vi "Actual Sample Mode.vi"(8 "error in (no error)":errorcluster {"code" format="%.0x"}, 11 "VISA Resource Name":refnum<visa-resource-name>) -> (0 "error out":errorcluster {"code" format="%.0x"}, 2 "Sample Mode":i32(ring)=1 items=["Real Time", "Equivalent Time"], 3 "VISA Resource Name Out":refnum<visa-resource-name>)   [LabVIEW 2010, in "Tektronix TDS 3000 Series.lvlib"]
doc: "This VI returns the sample mode the oscilloscope is currently using."
uses:
  <instrlib>/Tektronix TDS 3000 Series/Tektronix TDS 3000 Series.lvlib
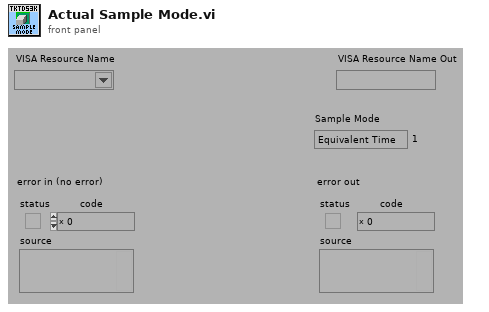
[diagram p1: front panel]
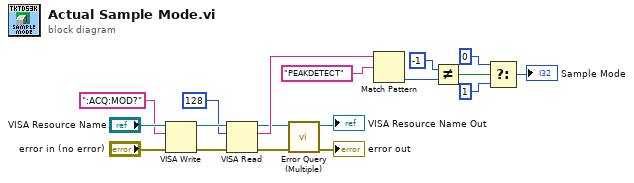
[diagram p0: block diagram]
diagram:
  n1 = VISA Write(VISA resource name="VISA Resource Name", write buffer=":ACQ:MOD?", error in (no error)="error in (no error)") -> (VISA resource name out=w18:refnum<visa-resource-name>, error out=w17:errorcluster)  [unwired: 1 out]
  n2 = VISA Read(VISA resource name=w18, byte count=u32 128, error in (no error)=w17) -> (VISA resource name out=w4:refnum<visa-resource-name>, read buffer=w12:string, error out=w3:errorcluster)  [unwired: 1 out]
  n3 = call <instrlib>:"Error Query (Multiple).vi"("error in (no error)"=w3, "VISA Resource Name"=w4) -> ("error out"=→"error out":errorcluster, "VISA Resource Name Out"=→"VISA Resource Name Out":refnum<visa-resource-name>)  [unwired: 6 in, 2 out]
  n4 = Match Pattern(string=w12, regular expression="PEAKDETECT") -> (offset past match=w10:i32)  [unwired: 1 in, 3 out]
  n5 = Not Equal?(x=-1, y=w10) -> (x != y?=w8:bool)
  n6 = Select(t=0, s=w8, f=1) -> (s? t:f=→"Sample Mode":i32)
